vi "add_3d_imaq_images.vi"(6 "error in":errorcluster, 8 "Images in 2":T1[](array[typedef]), 9 "Images in 1":T1[](array[typedef])) -> (0 "error out":errorcluster, 3 "Images out":T1[](array[typedef]))   [LabVIEW 2011, in "Fiberscope_library.lvlib"]
uses:
  Fiberscope_library.lvlib
  <vilib>/vision/Image Controls.llb/IMAQ Image.ctl
  <vilib>/vision/NI_Vision_Development_Module.lvlib
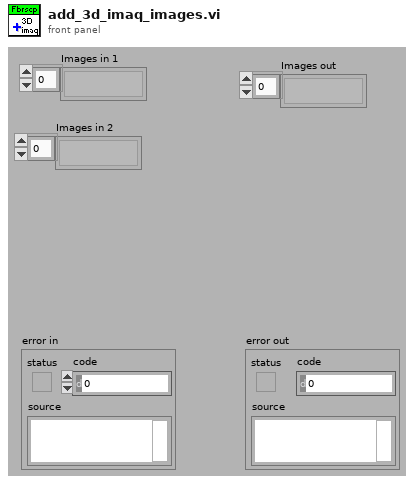
[diagram p1: front panel]
types:
  T1 = typedef "IMAQ Image.ctl" = refnum<image>
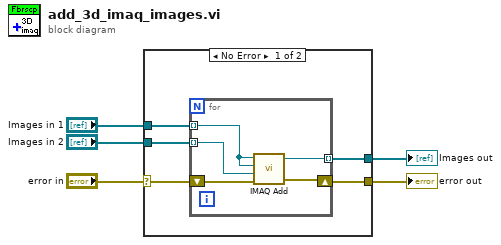
[diagram p0: block diagram]
diagram:
  n1 = case shown="No Error" "error in" {
    selector: "error in" -> [w8 w17]
    tunnel: [w7 w17] -> w4
    tunnel: "Images in 1" -> [w10 w16]
    tunnel: "Images in 2" -> [w9 _]
    tunnel: [w6 w16] -> w1
    frame No Error {
      n2 = for {
        tunnel: w10 -> [w12] mode=indexing
        tunnel: w9 -> [w13] mode=indexing
        shift-right: [w14] -> w7
        shift-left: w8 -> [w15]
        tunnel: [w11] -> w6 mode=indexing
        n3 = call "IMAQ Add"("Image Src A"=w12, "Image Dst"=w12, "Image Src B"=w13, "error in (no error)"=w15) -> ("Image Dst Out"=w11:T1, "error out"=w14:errorcluster)  [unwired: 3 in]
      }
    }
    frame Error {
    }
  }
  "error out" <- w4
  "Images out" <- w1
